vi "SR1.get data.vi"(0 "i ref in":refnum<vi>, 5 "error in (no error)":errorcluster) -> (14 "i ref out":refnum<vi>, 16 "Output Waveform":cluster{dbl, dbl, dbl[]}, 19 "error out":errorcluster)   [LabVIEW 2014, in "SR1.lvlib"]
doc: "gets the data in binary format from the SR1. The data format is a waveform."
uses:
  SR1.lvlib
  CS_Core/CSSystem/CoreDefs/CoreDefs.error_type.ctl
  CS_Core/CSSystem/CoreLib/CoreLib.lvlib
  CSlibraries/UtilityLib/UtilityLib.lvlib
  instr.lib/Stanford Research SR1/Stanford Research SR1.lvlib
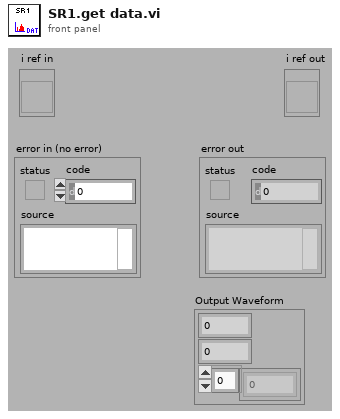
[diagram p1: front panel]
types:
  T1 = typedef "CoreDefs.error_type.ctl" = enum16{"no error", "can't load process", "can't unload process", "process does not exist", "can't install process", "can't remove process", "unknown function", "time out", "can't execute function", "duplicate queue name", "super not found", "caller queue invalid", "can't ping process", "unknown error", "VISA Error", "VISA timeout", "GPIB timeout", "GPIB error", "communication error", "data type mismatch", "can't read data from OPC server", "can't write data to OPC server", "OET error", "function not implemented", "process already exists", "invalid Shared Variable name", "error writing Shared Variable", "error reading Shared Variable", "invalid client name", "corrupt database", "unknown class", "call not authorized", "parameter out of range", "OET timeout: can't get data to modify", "invalid queue name", "requested operation incompatible with current state", "event undefined", "event disabled", "state undefined", "caller is not a friend", "EventBuilder: bad eventID", "EventBuilder: no DAQ devices", "a thread must not stop itself", "UNUSED ELEMENT4", "DiscArchiver: eventData incomplete", "DiscArchiver: eventData does not belong to run", "DiscArchiver: can't open file", "DiscArchiver: can't write to file", "DiscArchiver: available disc space low", "can't acquire semaphore", "error reading data from database", "notifier object is not existing", "can't register process", "can't unregister process", "illegal event type", "object disabled", "object already exists", "can't change state", "Instrument not found", "no connection to remote node", "invalid reference", "N/A", "UNUSED ELEMENT 1", "element not found", "illegal TCP/IP connection detected", "object does not exist", "invalid access ID", "unknown CS system", "invalid privilige", "unsupported data type", "unsupported server type", "IO server already exists", "Shared Variable already exists"}
  T2 = typedef "SR1.lvlib/SR1.i attribute.ctl" = cluster{"GraphID":i32, "TraceID":i32}
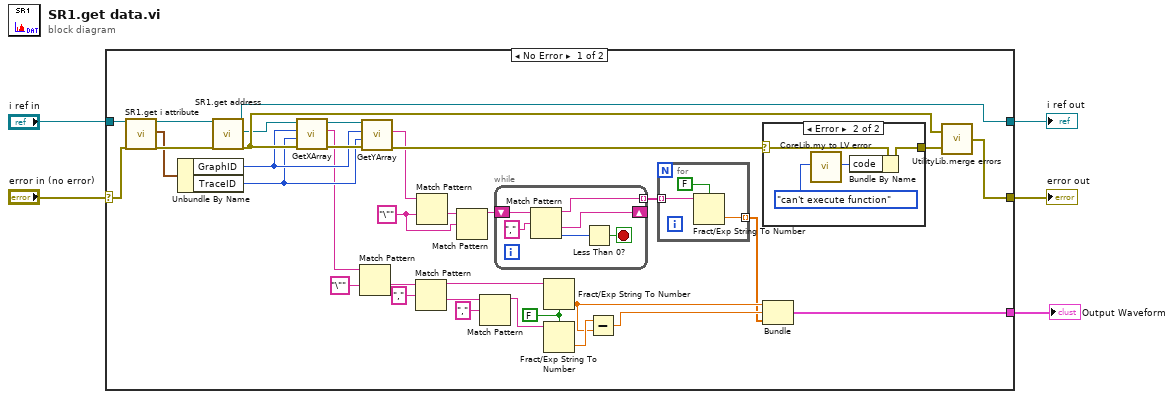
[diagram p0: block diagram]
diagram:
  n1 = case shown="No Error" "error in (no error)" {
    selector: "error in (no error)" -> [w6 w54]
    tunnel: "i ref in" -> [w7 w55]
    tunnel: [w38 w54] -> w4
    tunnel: [w39 w55] -> w3
    tunnel: [w37 _] -> w1
    frame No Error {
      w13 = "\"" ("regular expression")
      w18 = FALSE ("use system decimal point (T)")
      n2 = call "SR1.get i attribute.vi"("i ref in"=w7, "error in (no error)"=w6) -> ("i ref out"=w29:refnum<vi>, "i attribute"=w28:T2, "error out"=w30:errorcluster)  [unwired: 15 in]
      n3 = Unbundle By Name(w28) -> ("GraphID"=w27:i32, "TraceID"=w26:i32)
      n4 = call "SR1.get address.vi"("i ref in"=w29, "error in (no error)"=w30) -> ("i ref out"=w39:refnum<vi>, "VISA resource name"=w32:refnum<visa-resource-name>, "error out"=w35:errorcluster)  [unwired: 15 in]
      n5 = call "GetXArray.vi"("error in (no error)"=w35, "TraceID"=w26, "GraphID"=w27, "VISA resource name"=w32) -> ("error out"=w34:errorcluster, "xArray"=w16:string, "VISA resource name out"=w31:refnum<visa-resource-name>)  [unwired: 5 in]
      n6 = Match Pattern(string=w16, regular expression="\"") -> (after substring=w24:string)  [unwired: 1 in, 3 out]
      n7 = call "GetYArray.vi"("error in (no error)"=w34, "TraceID"=w26, "GraphID"=w27, "VISA resource name"=w31) -> ("error out"=w33:errorcluster, "yArray"=w9:string)  [unwired: 5 in, 1 out]
      n8 = Match Pattern(string=w24, regular expression=",") -> (before substring=w20:string, after substring=w21:string)  [unwired: 1 in, 2 out]
      n9 = Match Pattern(string=w9, regular expression=w13) -> (after substring=w11:string)  [unwired: 1 in, 3 out]
      n10 = Match Pattern(string=w11, regular expression=w13) -> (before substring=w12:string)  [unwired: 1 in, 3 out]
      n11 = Match Pattern(string=w21, regular expression=",") -> (before substring=w19:string)  [unwired: 1 in, 3 out]
      n12 = while {
        tunnel: [w43] -> w10 mode=indexing
        shift-right: [w42] -> _
        shift-left: w12 -> [w45]
        stop <- w40 stop-if-true
        n13 = Match Pattern(string=w45, regular expression=",") -> (before substring=w43:string, after substring=w42:string, offset past match=w41:i32)  [unwired: 1 in, 1 out]
        n14 = Less Than 0?(x=w41) -> (x < 0?=w40:bool)
      }
      n15 = Fract/Exp String To Number(use system decimal point (T)=w18, string=w20) -> (number=w14:dbl)  [unwired: 2 in, 1 out]
      n16 = Fract/Exp String To Number(use system decimal point (T)=w18, string=w19) -> (number=w17:dbl)  [unwired: 2 in, 1 out]
      n17 = Subtract(x=w17, y=w14) -> (x-y=w15:dbl)
      n18 = for {
        tunnel: w10 -> [w48] mode=indexing
        tunnel: [w46] -> w8 mode=indexing
        n19 = Fract/Exp String To Number(use system decimal point (T)=FALSE, string=w48) -> (number=w46:dbl)  [unwired: 2 in, 1 out]
      }
      n20 = case shown="Error" w33 {
        selector: w33 -> [w49 w53]
        tunnel: [w49 w50] -> w36
        frame No Error {
        }
        frame Error {
          n21 = call "CoreLib.my to LV error.vi"("ErrorTypes"=CoreDefs.error_type."can't execute function") -> ("LV error code"=w52:i32)  [unwired: 17 in, 1 out]
          n22 = Bundle By Name(cluster=w53, "code"=w52) -> (w50:errorcluster)
        }
      }
      n23 = Bundle(w14, w15, w8) -> (w37:cluster{dbl, dbl, dbl[]})  [unwired: 1 in]
      n24 = call "UtilityLib.merge errors.vi"("error2 (no error)"=w36, "error1 (no error)"=w35) -> ("error out"=w38:errorcluster)
    }
    frame Error {
    }
  }
  "error out" <- w4
  "i ref out" <- w3
  "Output Waveform" <- w1
